vi "Find Objects.vi"(0 "RowSum or ColSum":i16[](array[numeric]), 5 "error in (no error)":errorcluster, 7 "Threshhold":i32=100) -> (14 "Object(s) Start/Stop/Sum":i32[][](array[numeric]), 19 "error out":errorcluster)   [LabVIEW 2016]
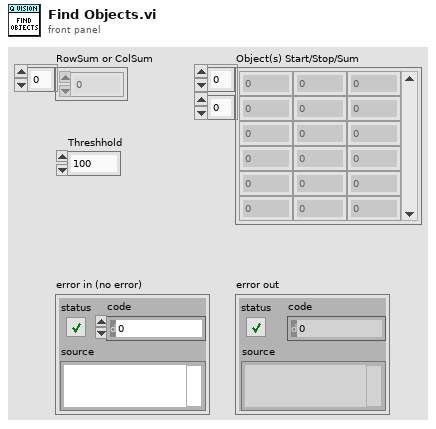
[diagram p1: front panel]
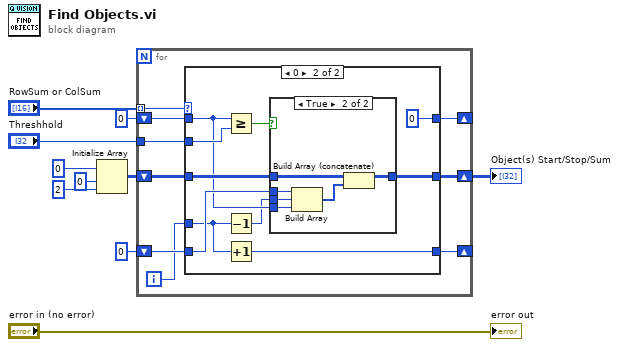
[diagram p0: block diagram]
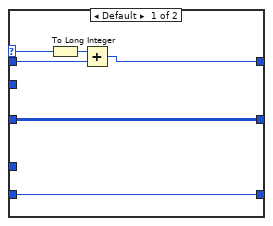
[diagram p2: hidden frame]
diagram:
  n1 = Initialize Array(0, 0 ("dimension size"), 2 ("dimension size")) -> (w8:i32[][])
  n2 = for {
    tunnel: "RowSum or ColSum" -> [w18] mode=indexing
    shift-right: [w17] -> _
    shift-left: 0 -> [w16]
    shift-right: [w13] -> w4
    shift-left: w8 -> [w19]
    shift-right: [w15] -> _
    shift-left: 0 -> [w14]
    tunnel: "Threshhold" -> [w12]
    i -> [w11]
    n3 = case shown="0" w18 {
      selector: w18 -> [w25 _]
      tunnel: w19 -> [w21 w33]
      tunnel: w11 -> [_ w30]
      tunnel: [w23 0] -> w17
      tunnel: w16 -> [w24 w28]
      tunnel: [w22 w27] -> w15
      tunnel: w14 -> [w22 w31]
      tunnel: [w21 w32] -> w13
      tunnel: w12 -> [_ w29]
      frame Default {
        n4 = To Long Integer(number=w25) -> (32bit integer=w20:i32)
        n5 = Add(x=w20, y=w24) -> (x+y=w23:i32)
      }
      frame 0 {
        n6 = Greater Or Equal?(x=w28, y=w29) -> (x >= y?=w34:bool)
        n7 = Decrement(x=w30) -> (x-1=w26:i32)
        n8 = Increment(x=w30) -> (x+1=w27:i32)
        n9 = case shown="True" w34 {
          tunnel: w33 -> [w36 w42]
          tunnel: [w36 w41] -> w32
          tunnel: w31 -> [_ w40]
          tunnel: w26 -> [_ w39]
          tunnel: w28 -> [_ w37]
          frame False {
          }
          frame True {
            n10 = Build Array(w40, w39, w37) -> (w38:i32[])
            n11 = Build Array (concatenate)(w42, w38) -> (w41:i32[][])
          }
        }
      }
    }
  }
  "Object(s) Start/Stop/Sum" <- w4
  "error out" <- "error in (no error)"
